vi "Test_AddUnnamedTopic_NoOpReturnError.vi"(8 "error in (no error)":errorcluster, 11 "TestCase in":refnum<class "TestTopicLookupTable.lvclass">) -> (0 "error out":errorcluster, 3 "TestCase out":refnum<class "TestTopicLookupTable.lvclass">)   [LabVIEW 2017, in "TestTopicLookupTable.lvclass"]
uses:
  TestTopicLookupTable.lvclass
  gpm_packages/@cs/event-logger/Source/Composed Log/LoggerReference/LoggerReference.lvclass
  <vilib>/ActorFramework/Message Queue/Message Queue.lvclass/Message Queue.ctl
  Source/Framework/Mediator/Topic/Topic.lvclass/Topic.ctl
  Source/Framework/Mediator/TopicLookupTable/TopicLookupTable.lvclass/TopicLookupTable.ctl
  Source/Framework/Mediator/Topic/Read Topic Info.vi
  <vilib>/ActorFramework/Actor/Read Self Enqueuer.vi
  <vilib>/ActorFramework/Message Enqueuer/Init from Existing Queue.vi
  gpm_packages/@cs/variant/Source/Format Type String.vi
  Source/Framework/Mediator/Topic/Topic.lvclass
  <vilib>/ActorFramework/Message Enqueuer/Message Enqueuer.lvclass
  Source/Framework/Mediator/TopicLookupTable/TopicLookupTable.lvclass
  <vilib>/ActorFramework/Message Queue/Message Queue.lvclass
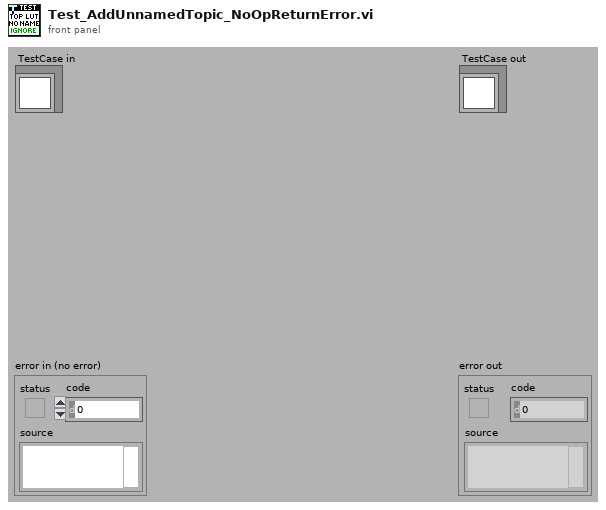
[diagram p1: front panel]
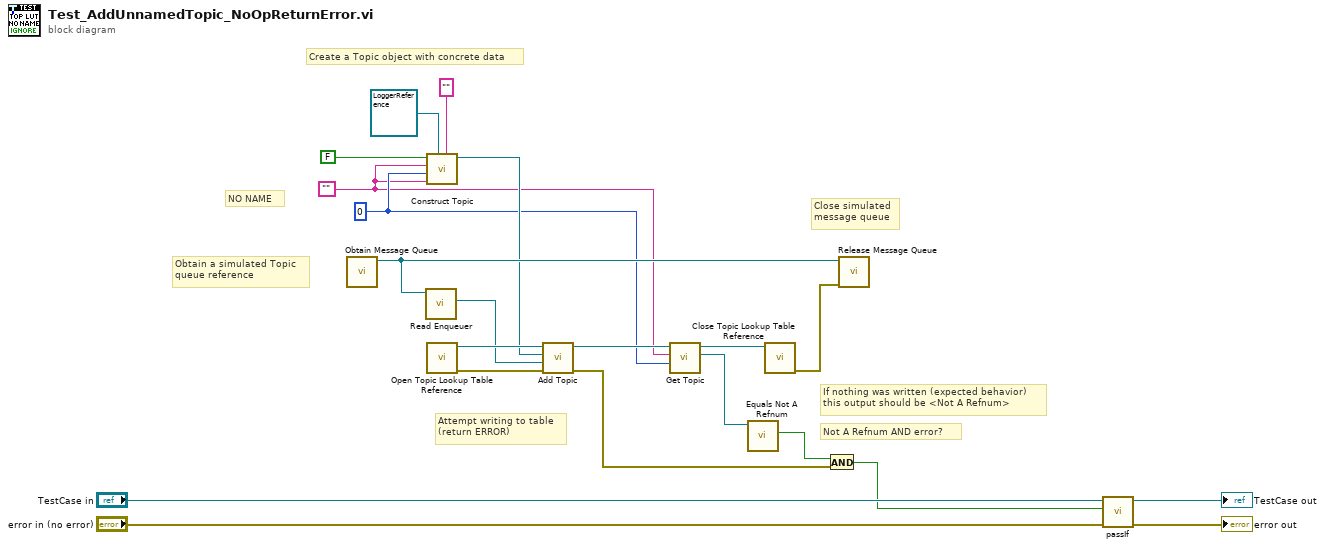
[diagram p0: block diagram]
diagram:
  w8 = 0
  w3 = "" ("Name")
  # "Not A Refnum AND error?"
  # "If nothing was written (expected behavior)\nthis output should be <Not A Refnum>"
  # "NO NAME"
  # "Create a Topic object with concrete data"
  # "Attempt writing to table\n(return ERROR)"
  # "Close simulated\nmessage queue"
  # "Obtain a simulated Topic\nqueue reference"
  n1 = call <vilib>:"Obtain Message Queue.vi"() -> ("Message Queue"=w12:refnum<class "Message Queue.lvclass">)  [unwired: 10 in, 1 out]
  n2 = call <vilib>:"Read Enqueuer.vi"("Message Queue"=w12) -> ("Message Enqueuer"=w14:refnum<class "Message Enqueuer.lvclass">)  [unwired: 10 in]
  n3 = call "Construct Topic.vi"("Framework Instance Alias"="", "Event Log Instance"=refnum<class "LoggerReference.lvclass"> refnum, "Lock Owner ID (\"\" = NOT Locked)"=w3, "New Topic Data"=w8, "Name"=w3, "Use Type Input As Initial Value?"=FALSE) -> ("Topic out"=w10:refnum<class "Topic.lvclass">)  [unwired: 4 in, 1 out]
  n4 = call "Open Topic Lookup Table Reference.vi"() -> ("error out"=w16:errorcluster, "TopicLookupTable Reference"=w17:refnum<data-value>)  [unwired: 10 in]
  n5 = call "Add Topic.vi"("error in (no error)"=w16, "Topic Enqueuer"=w14, "Topic Object"=w10, "TopicLookupTable"=w17) -> ("error out"=w5:errorcluster, "TopicLookupTable"=w15:refnum<data-value>)  [unwired: 5 in, 1 out]
  n6 = call "Get Topic.vi"("Topic Type"=w8, "Topic Name"=w3, "TopicLookupTable"=w15) -> ("Topic Enqueuer"=w7:refnum<class "Message Enqueuer.lvclass">, "TopicLookupTable"=w9:refnum<data-value>)  [unwired: 6 in, 1 out]
  n7 = call <vilib>:"Equals Not A Refnum.vi"("Message Enqueuer"=w7) -> ("Not a refnum?"=w6:bool)  [unwired: 10 in]
  n8 = call "Close Topic Lookup Table Reference.vi"("TopicLookupTable"=w9) -> ("error out"=w13:errorcluster)  [unwired: 10 in]
  n9 = And(x=w6, y=w5) -> (x .and. y?=w4:bool)
  n10 = call <vilib>:"Release Message Queue.vi"("error in (no error)"=w13, "Message Queue"=w12) -> ()  [unwired: 8 in, 2 out]
  n11 = call-dynamic "passIf.vi"("error in (no error)"="error in (no error)", "pass"=w4, "TestCase in"="TestCase in") -> ("error out"=→"error out":errorcluster, "TestCase out"=→"TestCase out":refnum<class "TestTopicLookupTable.lvclass">)  [unwired: 7 in]
